vi "tcs shm issue Command wfp Simulate LV.vi"(8 "error in (no error)":errorcluster, 11 "command_wfpSimulate_Ctl":T1) -> (0 "error out":errorcluster, 2 "function return":i32, 3 "command_wfpSimulate_Ctl out":T1)   [LabVIEW 2016, in "SALLV_tcs.lvlib"]
doc: "int tcs_shm_issueCommand_wfpSimulateLV(tcs_command_wfpSimulateLV *command_wfpSimulate_Ctl );"
uses:
  SALLV_tcs.lvlib
  SALLV_tcs.so
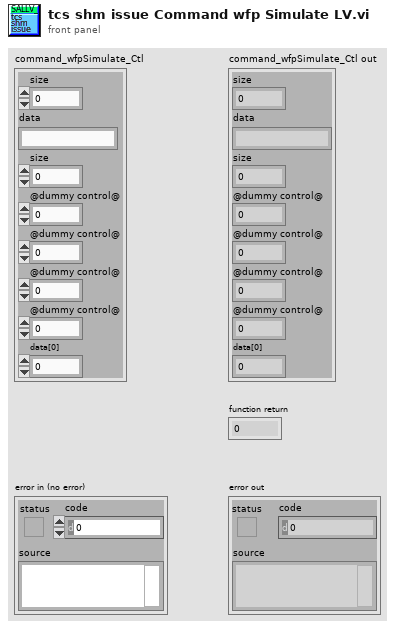
[diagram p1: front panel]
types:
  T1 = cluster{"size":i32, "data":string, "size":i32, "@dummy control@":i8, "@dummy control@":i8, "@dummy control@":i8, "@dummy control@":i8, "data[0]":dbl}
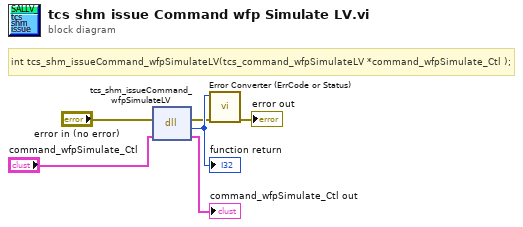
[diagram p0: block diagram]
diagram:
  # "int tcs_shm_issueCommand_wfpSimulateLV(tcs_command_wfpSimulateLV *command_wfpSimulate_Ctl );"
  n1 = dll-call lib="home/andres/Desktop/SALLV_tcs/SALLV_tcs.*" fn="tcs_shm_issueCommand_wfpSimulateLV"(error in="error in (no error)", "command_wfpSimulate_Ctl"="command_wfpSimulate_Ctl") -> (error out=w2:errorcluster, w6:i32, "command_wfpSimulate_Ctl"=→"command_wfpSimulate_Ctl out":T1)  [unwired: 2 in, 1 out]
  "function return" <- w6
  n2 = call "Error Converter (ErrCode or Status).vi"("error in (no error)"=w2, "error code"=w6) -> ("error out"=→"error out":errorcluster)  [unwired: 9 in]
